vi "FXP NIPLL_AveragingPD.vi"(6 "alpha [U16.0]":fxp<+,16,0>, 8 "sin(z) [I16.2]":fxp<+/-,16,2> format="%.23g", 9 "cos(z) [I16.2]":fxp<+/-,16,2> format="%.23g", 11 "x[I16.1]":fxp<+/-,16,1>) -> (3 "psd_out":fxp<+/-,16,2> format="%.15g")   [LabVIEW 2009]
uses:
  <vilib>/rvi/FXPMathLib/FxpMul/XNode/nifxpmath_Multiplier.xnode
  <vilib>/rvi/FXPMathLib/FxpMul/subVIs/nifxpmath_Mul_SimConfig.ctl
  <vilib>/fxp/LVFixedPointQuantizationPolicyTypeDef.ctl
  <vilib>/fxp/LVFixedPointOverflowPolicyTypeDef.ctl
  <vilib>/rvi/FXPMathLib/FxpMul/simVIs/DllFxpMulTemp_sub.vi
  <vilib>/rvi/FXPMathLib/FxpConvert/XNode/nifxpmath_Convert.xnode
  <vilib>/rvi/FXPMathLib/FxpConvert/subVIs/nifxpmath_Convert_SimConfig.ctl
  <vilib>/rvi/FXPMathLib/FxpConvert/simVIs/DllFxpConvertTemp_sub.vi
  <vilib>/rvi/FXPMathLib/FxpAtan2/XNode/nifxpmath_Atan2.xnode
  <vilib>/rvi/FXPMathLib/FxpAtan2/subVIs/nifxpmath_Atan2_SimConfig.ctl
  <vilib>/rvi/FXPMathLib/FxpAtan2/simVIs/DllFxpAtan2Temp_sub.vi
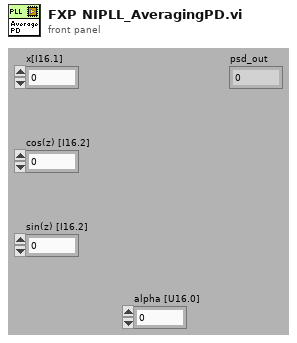
[diagram p1: front panel]
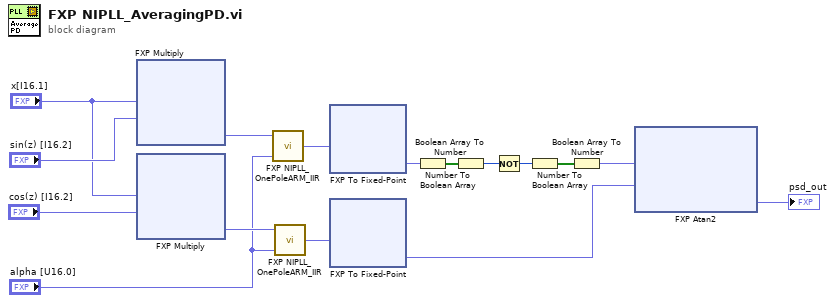
[diagram p0: block diagram]
diagram:
  n1 = xnode "FXP Multiply"("x"="x[I16.1]", "y"="sin(z) [I16.2]") -> ("x*y"=w16:fxp<+/-,32,3>)
  n2 = xnode "FXP Multiply"("x"="x[I16.1]", "y"="cos(z) [I16.2]") -> ("x*y"=w15:fxp<+/-,32,3>)
  n3 = call "FXP NIPLL_OnePoleARM_IIR.vi"("alpha [U16.0]"="alpha [U16.0]", "x"=w16) -> ("y[n]"=w9:fxp<+/-,48,3>)  [unwired: 1 in]
  n4 = call "FXP NIPLL_OnePoleARM_IIR.vi"("alpha [U16.0]"="alpha [U16.0]", "x"=w15) -> ("y[n]"=w8:fxp<+/-,48,3>)  [unwired: 1 in]
  n5 = xnode "FXP To Fixed-Point"("x"=w9) -> ("y"=w7:fxp<+/-,32,3>)
  n6 = xnode "FXP To Fixed-Point"("x"=w8) -> ("y"=w1:fxp<+/-,32,3>)
  n7 = Number To Boolean Array(number=w7) -> (Boolean array=w6:bool[])
  n8 = Boolean Array To Number(Boolean array=w6) -> (number=w5:u32)
  n9 = Not(x=w5) -> (.not. x?=w4:u32)
  n10 = Number To Boolean Array(number=w4) -> (Boolean array=w3:bool[])
  n11 = Boolean Array To Number(Boolean array=w3) -> (number=w2:fxp<+/-,32,3>)
  n12 = xnode "FXP Atan2"("y"=w2, "x"=w1) -> ("atan2(y,x) (pi)"=→"psd_out":fxp<+/-,16,2>)
